vi "async safe state action.vi"(0 "output to component":refnum<queue>, 2 "system error in":errorcluster, 3 "execution settings":T1, 5 "output from component":refnum<queue>, 7 "process input to component":refnum<queue>, 9 "process result to component":refnum<queue>, 11 "process input from component":refnum<queue>, 12 "process result from component":refnum<queue>, 13 "module in":refnum<class "TBM module execution interface.lvclass">, 14 "module error in":errorcluster) -> (4 "system error out":errorcluster, 10 "module out":refnum<class "TBM module execution interface.lvclass">, 15 "module error out":errorcluster)   [LabVIEW 2013, in "Standard Engine Runtime.lvclass"]
uses:
  Standard Engine Runtime.lvclass
  <vilib>/NI/Tag Bus Module Framework/runtime/TBM module execution interface.lvclass
  <vilib>/NI/Tag Bus Module Framework/runtime/execution settings.ctl
  <vilib>/NI/Tag Bus/table/data table.ctl
  <vilib>/NI/Tag Bus/table/data table.lvlib
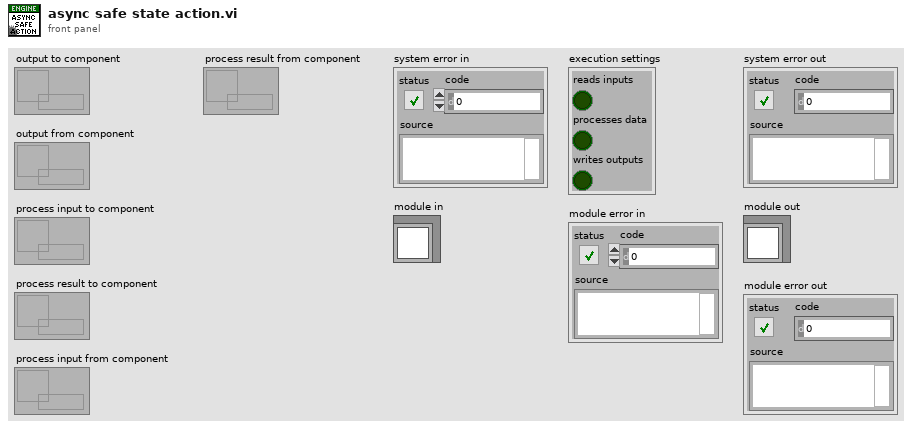
[diagram p1: front panel]
types:
  T1 = typedef "TBM module execution interface.lvclass/execution settings.ctl" = cluster{"reads inputs":bool, "processes data":bool, "writes outputs":bool}
  T2 = typedef "tag bus.lvlib/data table.lvlib/data table.ctl" = cluster{"Double":dbl[], "Single":sgl[], "I64":i64[], "I32":i32[], "I16":i16[], "I8":i8[], "U64":u64[], "U32":u32[], "U16":u16[], "U8":u8[], "Boolean":bool[], "String":string[], "Array of Double":cluster{"DBL Array":dbl[]}[], "Array of Single":cluster{"SGL Array":sgl[]}[], "Array of I64":cluster{"I64 Array":i64[]}[], "Array of I32":cluster{"I32 Array":i32[]}[], "Array of I16":cluster{"I16 Array":i16[]}[], "Array of I8":cluster{"I8 Array":i8[]}[], "Array of U64":cluster{"U64 Array":u64[]}[], "Array of U32":cluster{"U32 Array":u32[]}[], "Array of U16":cluster{"U16 Array":u16[]}[], "Array of U8":cluster{"U8 Array":u8[]}[], "Array of Boolean":cluster{"Boolean Array":bool[]}[], "Array of String":cluster{"String Array":string[]}[]}
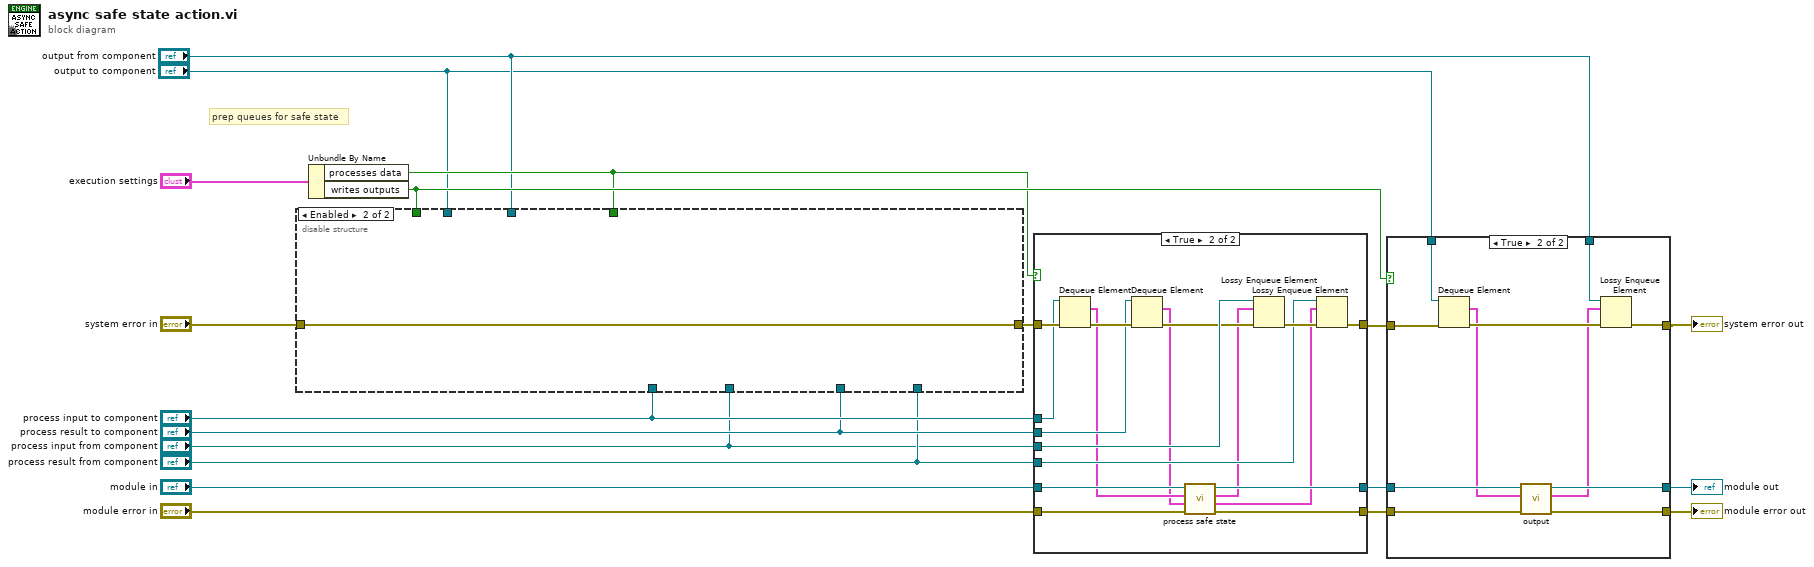
[diagram p0: block diagram]
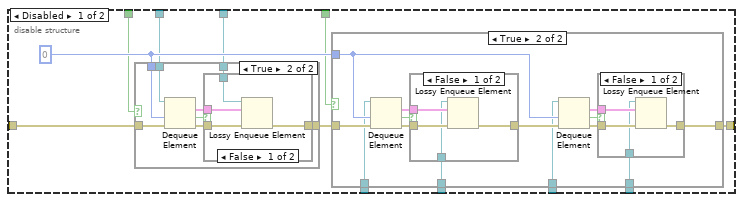
[diagram p2: hidden frame]
diagram:
  # "prep queues for safe state"
  n1 = Unbundle By Name("execution settings") -> ("processes data"=w16:bool, "writes outputs"=w17:bool)
  n2 = disable-structure shown="Enabled" {
    disable-tunnel: "system error in" -> [w31 w71]
    disable-tunnel: w17 -> [w28 _]
    disable-tunnel: w16 -> [w27 _]
    disable-tunnel: [w26 w71] -> w7
    disable-tunnel: "output from component" -> [w25 _]
    disable-tunnel: "output to component" -> [w24 _]
    disable-tunnel: "process input to component" -> [w23 _]
    disable-tunnel: "process result to component" -> [w22 _]
    disable-tunnel: "process result from component" -> [w21 _]
    disable-tunnel: "process input from component" -> [w20 _]
    frame Disabled {
      w29 = 0 ("timeout in ms (-1)")
      n3 = case shown="True" w28 {
        tunnel: w31 -> [w57 w65]
        tunnel: w24 -> [_ w64]
        tunnel: w25 -> [_ w62]
        tunnel: [w57 w59] -> w30
        tunnel: w29 -> [_ w58]
        frame False {
        }
        frame True {
          n4 = Dequeue Element(queue=w64, timeout in ms (-1)=w58, error in (no error)=w65) -> (element=w61:T2, timed out?=w60:bool, error out=w63:errorcluster)  [unwired: 1 out]
          n5 = case shown="False" w60 {
            tunnel: w63 -> [w69 w70]
            tunnel: w62 -> [w68 _]
            tunnel: w61 -> [w67 _]
            tunnel: [w66 w70] -> w59
            frame False {
              n6 = Lossy Enqueue Element(queue=w68, element=w67, error in (no error)=w69) -> (error out=w66:errorcluster)  [unwired: 3 out]
            }
            frame True {
            }
          }
        }
      }
      n7 = case shown="True" w27 {
        tunnel: w30 -> [w32 w40]
        tunnel: w29 -> [_ w38]
        tunnel: w23 -> [_ w37]
        tunnel: w22 -> [_ w36]
        tunnel: w20 -> [_ w35]
        tunnel: w21 -> [_ w34]
        tunnel: [w32 w33] -> w26
        frame False {
        }
        frame True {
          n8 = Dequeue Element(queue=w37, timeout in ms (-1)=w38, error in (no error)=w40) -> (element=w45:T2, timed out?=w46:bool, error out=w44:errorcluster)  [unwired: 1 out]
          n9 = case shown="False" w46 {
            tunnel: w44 -> [w55 w56]
            tunnel: w45 -> [w54 _]
            tunnel: [w53 w56] -> w39
            tunnel: w35 -> [w52 _]
            frame False {
              n10 = Lossy Enqueue Element(queue=w52, element=w54, error in (no error)=w55) -> (error out=w53:errorcluster)  [unwired: 3 out]
            }
            frame True {
            }
          }
          n11 = Dequeue Element(queue=w36, timeout in ms (-1)=w38, error in (no error)=w39) -> (element=w42:T2, timed out?=w41:bool, error out=w43:errorcluster)  [unwired: 1 out]
          n12 = case shown="False" w41 {
            tunnel: w43 -> [w50 w51]
            tunnel: w42 -> [w49 _]
            tunnel: [w48 w51] -> w33
            tunnel: w34 -> [w47 _]
            frame False {
              n13 = Lossy Enqueue Element(queue=w47, element=w49, error in (no error)=w50) -> (error out=w48:errorcluster)  [unwired: 3 out]
            }
            frame True {
            }
          }
        }
      }
    }
    frame Enabled {
    }
  }
  n14 = case shown="True" w16 {
    tunnel: "module in" -> [w74 w82]
    tunnel: [w74 w80] -> w14
    tunnel: [w73 w81] -> w13
    tunnel: "module error in" -> [w73 w83]
    tunnel: [w72 w87] -> w8
    tunnel: w7 -> [w72 w91]
    tunnel: "process input to component" -> [_ w90]
    tunnel: "process result to component" -> [_ w88]
    tunnel: "process result from component" -> [_ w85]
    tunnel: "process input from component" -> [_ w84]
    frame False {
    }
    frame True {
      n15 = Dequeue Element(queue=w90, error in (no error)=w91) -> (element=w76:T2, error out=w89:errorcluster)  [unwired: 1 in, 2 out]
      n16 = Dequeue Element(queue=w88, error in (no error)=w89) -> (element=w75:T2, error out=w79:errorcluster)  [unwired: 1 in, 2 out]
      n17 = call-dynamic "process safe state.vi"("error in"=w83, "result allocation"=w75, "parameters"=w76, "module in"=w82) -> ("error out"=w81:errorcluster, "results"=w77:T2, "parameter allocation"=w78:T2, "module out"=w80:refnum<class "TBM module execution interface.lvclass">)  [unwired: 4 in]
      n18 = Lossy Enqueue Element(queue=w84, element=w78, error in (no error)=w79) -> (error out=w86:errorcluster)  [unwired: 3 out]
      n19 = Lossy Enqueue Element(queue=w85, element=w77, error in (no error)=w86) -> (error out=w87:errorcluster)  [unwired: 3 out]
    }
  }
  n20 = case shown="True" w17 {
    tunnel: w14 -> [w93 w100]
    tunnel: w13 -> [w94 w96]
    tunnel: [w94 w95] -> w11
    tunnel: [w93 w99] -> w10
    tunnel: [w92 w104] -> w9
    tunnel: w8 -> [w92 w103]
    tunnel: "output from component" -> [_ w101]
    tunnel: "output to component" -> [_ w102]
    frame False {
    }
    frame True {
      n21 = Dequeue Element(queue=w102, error in (no error)=w103) -> (element=w97:T2, error out=w105:errorcluster)  [unwired: 1 in, 2 out]
      n22 = call-dynamic "output.vi"("error in"=w96, "output data"=w97, "module in"=w100) -> ("error out"=w95:errorcluster, "output allocation"=w98:T2, "module out"=w99:refnum<class "TBM module execution interface.lvclass">)  [unwired: 6 in]
      n23 = Lossy Enqueue Element(queue=w101, element=w98, error in (no error)=w105) -> (error out=w104:errorcluster)  [unwired: 3 out]
    }
  }
  "module error out" <- w11
  "module out" <- w10
  "system error out" <- w9
